vi "As PropertyObjectFile.vi"(8 "error in (no error)":errorcluster, 11 "PropertyObjectFile in":refnum<class "PropertyObjectFile.lvclass">) -> (0 "error out":errorcluster, 2 "PropertyObjectFile":refnum<k7>, 3 "PropertyObjectFile out":refnum<class "PropertyObjectFile.lvclass">)   [LabVIEW 2020, in "TSnax.lvlib" / "PropertyObjectFile.lvclass"]
uses:
  PropertyObjectFile.lvclass
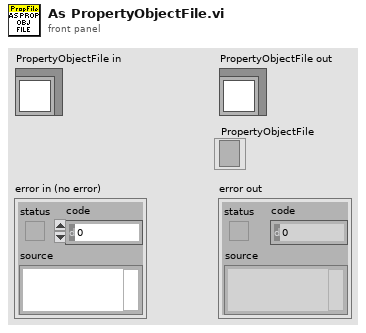
[diagram p1: front panel]
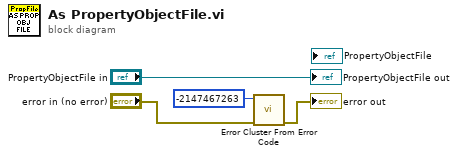
[diagram p0: block diagram]
diagram:
  n1 = call <vilib>:"Error Cluster From Error Code.vi"("error in (no error)"="error in (no error)", "error code (0)"=-2147467263) -> ("error out"=→"error out":errorcluster)  [unwired: 7 in]
  "PropertyObjectFile out" <- "PropertyObjectFile in"
